vi "xyzd2vector.vi"(1 "offset":cluster{"x":i32, "y":i32}={"x"=100, "y"=100}, 2 "xyzd":dbl[](array[numeric])=[0.0, 0.0, 0.0, 1.0]) -> (0 "vector":cluster{"x":dbl, "y":dbl})   [LabVIEW 2011]
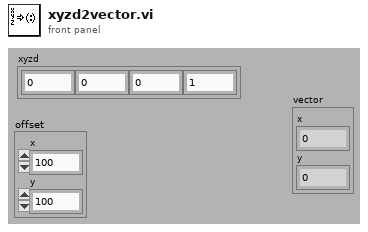
[diagram p1: front panel]
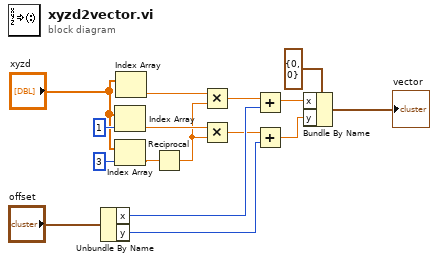
[diagram p0: block diagram]
diagram:
  n1 = Unbundle By Name("offset") -> ("x"=w15:i32, "y"=w16:i32)
  n2 = Index Array(array="xyzd", index=1) -> (element=w3:dbl)
  n3 = Index Array(array="xyzd", index=3) -> (element=w1:dbl)
  n4 = Index Array(array="xyzd") -> (element=w6:dbl)  [unwired: 1 in]
  n5 = Reciprocal(x=w1) -> (1/x=w2:dbl)
  n6 = Multiply(x=w6, y=w2) -> (x*y=w5:dbl)
  n7 = Multiply(x=w3, y=w2) -> (x*y=w4:dbl)
  n8 = Add(x=w5, y=w15) -> (x+y=w12:dbl)
  n9 = Add(x=w4, y=w16) -> (x+y=w11:dbl)
  n10 = Bundle By Name(cluster=cluster{"x":i16, "y":i16} {"x"=0, "y"=0}, "x"=w12, "y"=w11) -> (→"vector":cluster{"x":i16, "y":i16})
